vi "GFL Config Parse Results.vi"(0 "Previous Pass/Fail":bool=TRUE, 5 "Previous Report Text":string, 7 "found?":bool, 9 "key":string="Tester", 11 "section":string="Report Header") -> (4 "Pass/Fail":bool, 6 "Report Text":string)   [LabVIEW 2016]
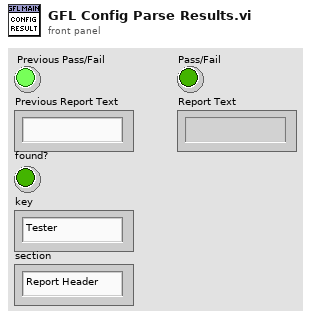
[diagram p1: front panel]
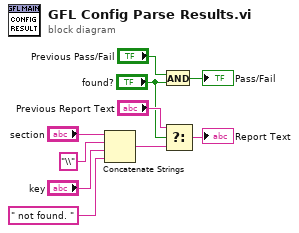
[diagram p0: block diagram]
diagram:
  n1 = Concatenate Strings("section", "\\" ("string"), "key", " not found. " ("string")) -> (w8:string)
  n2 = And(x="Previous Pass/Fail", y="found?") -> (x .and. y?=→"Pass/Fail":bool)
  n3 = Select(t="Previous Report Text", s="found?", f=w8) -> (s? t:f=→"Report Text":string)
